vi "SubVI DB.vi"(6 "Numeric":i32, 8 "Empresa":string, 9 "Area":string, 10 "Nombre":string) -> (0 "Numeric 2":i32)   [LabVIEW 2019, in "Base de datos.lvlib"]
uses:
  Base de datos.lvlib
  <vilib>/drjdpowell/SQLite Library/SQL Statement/SQL Statement.lvclass/SQL Statement.ctl
  <vilib>/drjdpowell/SQLite Library/SQL Connection/Open (path).vi
  <vilib>/drjdpowell/SQLite Library/SQL Statement/Bind Text.vi
  <vilib>/drjdpowell/SQLite Library/SQL Connection/Open (string).vi
  <vilib>/drjdpowell/SQLite Library/SQL Statement/Step.vi
  <vilib>/AdvancedString/Path To Command Line String.vi
  <vilib>/drjdpowell/SQLite Library/SQL Connection/Execute SQL (Single Integer).vi
  <vilib>/drjdpowell/SQLite Library/SQL Statement/Error Message.vi
  <vilib>/drjdpowell/SQLite Library/SQL Connection/Connection.lvclass
  <vilib>/drjdpowell/SQLite Library/SQLite.lvlib
  <vilib>/drjdpowell/SQLite Library/SQL Statement/SQL Statement.lvclass
  <vilib>/drjdpowell/SQLite Library/Transaction Helpers/Transaction.lvlib
  Config/Config.lvlib
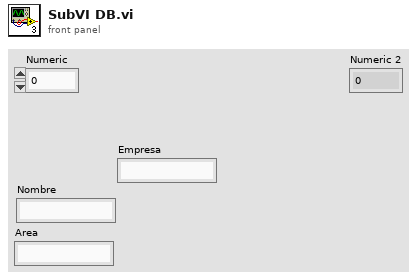
[diagram p1: front panel]
types:
  T1 = enum16{"New or existing", "Existing", "Read only"}
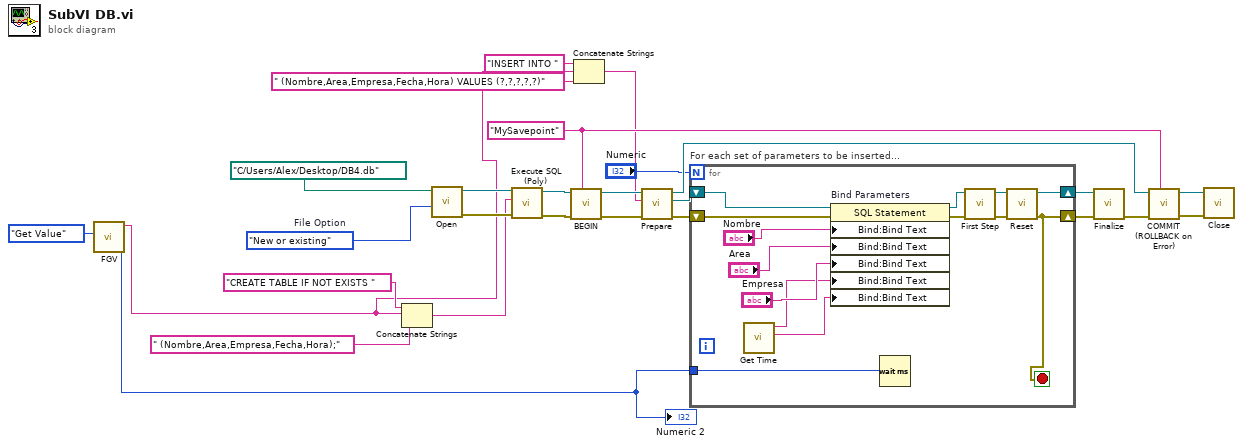
[diagram p0: block diagram]
diagram:
  w22 = "MySavepoint" ("Savepoint name")
  w25 = T1."New or existing"  # File Option
  n1 = call "FGV.vi"("Function"=enum16{"Set Value", "Get Value"}."Get Value") -> ("Numeric 2"=w1:i32, "Value out"=w2:string)  [unwired: 9 in]
  "Numeric 2" <- w1
  n2 = Concatenate Strings("CREATE TABLE IF NOT EXISTS " ("SQL"), w2, " (Nombre,Area,Empresa,Fecha,Hora);" ("string")) -> (w8:string)
  n3 = call-poly <vilib>:"Open.vi"("File Option"=w25, "db file"=path "C:/Users/Alex/Desktop/DB4.db") -> ("error out"=w27:errorcluster, "SQLite Connection"=w26:refnum<class "Connection.lvclass">)  [unwired: 8 in]
  n4 = call-poly <vilib>:"Execute SQL (Poly).vi"("error in (no error)"=w27, "SQL"=w8, "SQLite Connection in"=w26) -> ("error out"=w14:errorcluster, "SQLite Connection"=w15:refnum<class "Connection.lvclass">)  [unwired: 6 in, 1 out]
  n5 = call <vilib>:"BEGIN.vi"("Savepoint name"=w22, "error in (no error)"=w14, "SQLite Connection in"=w15) -> ("error out"=w21:errorcluster, "SQLite Connection"=w20:refnum<class "Connection.lvclass">)  [unwired: 7 in]
  n6 = Concatenate Strings("INSERT INTO " ("string"), w2, " (Nombre,Area,Empresa,Fecha,Hora) VALUES (?,?,?,?,?)" ("string")) -> (w7:string)
  n7 = call <vilib>:"Prepare.vi"("error in (no error)"=w21, "SQL"=w7, "SQLite Connection in"=w20) -> ("error out"=w17:errorcluster, "SQL Statement"=w16:refnum<class "SQL Statement.lvclass">, "SQLite Connection"=w23:refnum<class "Connection.lvclass">)  [unwired: 4 in, 2 out]
  n8 = for "For each set of parameters to be inserted..." {
    N: "Numeric" -> [_]
    shift-right: [w35] -> w18
    shift-left: w16 -> [w41]
    shift-right: [w29] -> w19
    shift-left: w17 -> [w38]
    tunnel: w1 -> [w28]
    stop <- w29 stop-if-true
    n9 = call "Get Time.vi"() -> ("Hora"=w31:string, "Fecha"=w30:string)  [unwired: 10 in]
    n10 = property on="Bind Parameters" class="SQL Statement"(reference=w41, error in=w38, "Bind:Bind Text"="Nombre", "Bind:Bind Text"="Area", "Bind:Bind Text"="Empresa", "Bind:Bind Text"=w30, "Bind:Bind Text"=w31) -> (reference out=w40:refnum<class "SQL Statement.lvclass">, error out=w39:errorcluster)
    n11 = Wait (ms)(milliseconds to wait=w28) -> ()  [unwired: 1 out]
    n12 = call <vilib>:"First Step.vi"("error in (no error)"=w39, "SQL Statement in"=w40) -> ("error out"=w37:errorcluster, "SQL Statement"=w36:refnum<class "SQL Statement.lvclass">)  [unwired: 7 in, 1 out]
    n13 = call <vilib>:"Reset.vi"("error in (no error)"=w37, "SQL Statement in"=w36) -> ("error out"=w29:errorcluster, "SQL Statement"=w35:refnum<class "SQL Statement.lvclass">)  [unwired: 8 in]
  }
  n14 = call <vilib>:"Finalize.vi"("error in (no error)"=w19, "SQL Statement in"=w18) -> ("error out"=w24:errorcluster)  [unwired: 9 in]
  n15 = call <vilib>:"COMMIT (ROLLBACK on Error).vi"("Savepoint name"=w22, "error in (no error)"=w24, "SQLite Connection in"=w23) -> ("error out"=w12:errorcluster, "SQLite Connection"=w13:refnum<class "Connection.lvclass">)  [unwired: 7 in]
  n16 = call-dynamic "Close.vi"("error in (no error)"=w12, "SQLite Connection in"=w13) -> ()  [unwired: 9 in, 1 out]
